vi "GetFaultListConv.vi"(2 "Fault message":u8 format="%x") -> (0 "Fault list":string)   [LabVIEW 2017]
panel:
  in  "Fault string":string[](array[string])=["Bad command", "Bad Id setpoint", "Bad Iq setpoint", "sqrt(I^2+Iq^2) violation", "Bad Isrc violation", "Bad Vsrc violation", "Bad V setpoint", "Bad f setpoint"]
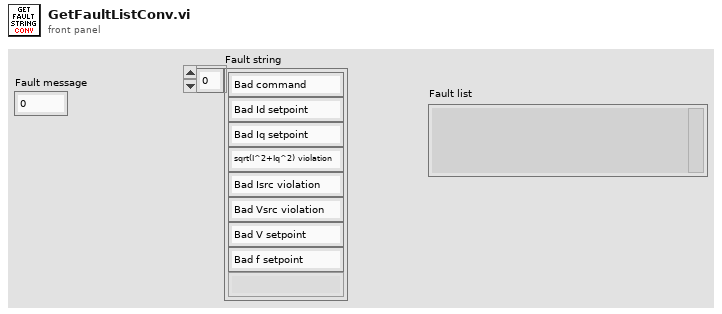
[diagram p1: front panel]
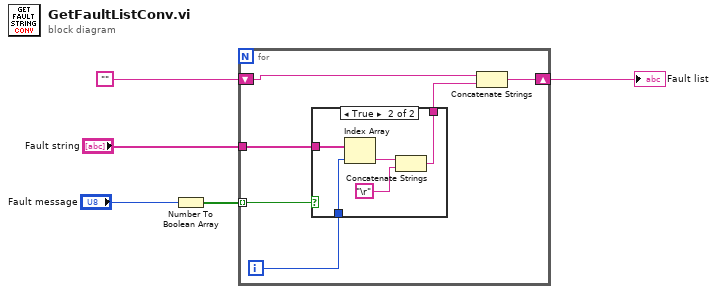
[diagram p0: block diagram]
diagram:
  n1 = Number To Boolean Array(number="Fault message") -> (Boolean array=w1:bool[])
  n2 = for {
    tunnel: "Fault string" -> [w11]
    tunnel: w1 -> [w10] mode=indexing
    shift-right: [w8] -> w5
    shift-left: "" -> [w9]
    i -> [w6]
    n3 = case shown="True" w10 {
      tunnel: w11 -> [_ w13]
      tunnel: w6 -> [_ w16]
      tunnel: [_ w14] -> w7
      frame False {
      }
      frame True {
        n4 = Index Array(array=w13, index=w16) -> (element=w12:string)
        n5 = Concatenate Strings(w12, "\r") -> (w14:string)
      }
    }
    n6 = Concatenate Strings(w9, w7) -> (w8:string)
  }
  "Fault list" <- w5
